vi "Hardware-EPTxControlCalPoints.vi"() -> (1 "EPTx Settings File Path":string, 3 "LoadEPTx Settings":bool, 4 "EPTxState":T4, 6 "EPTx Signal Select":T2, 8 "EPTxFilters":T3 {"Aux 4 [s]" format="%#_6p"; "Aux 3 [s]" format="%#_6p"; "Aux 2 [s]" format="%#_6p"; "Aux 1 [s]" format="%#_6p"; "Primary [s]" format="%#_6p"}, 10 "StallSpeed [RPM]":sgl, 15 "HistoryCAD":u8)   [LabVIEW 2016, in "DSI-RT.lvlib"]
uses:
  DSI-RT.lvlib
  <vilib>/Powertrain Controls/Device Drivers/Engine Position Tracking/EPTx/RevA/RT/Controls/EPTxState.ctl
  <vilib>/Powertrain Controls/Device Drivers/Engine Position Tracking/EPTx/RevA/RT/Controls/EPTxFilters.ctl
  <vilib>/Powertrain Controls/Device Drivers/DCM/Rev0/FPGA/Digital Channel.ctl
  <vilib>/addons/Software Calibration Management/xSCM/CalPoint.xnode
  <vilib>/Powertrain Controls/Device Drivers/Engine Position Tracking/EPTx/RevA/RT/EPTx - RevA - RT.lvlib
  <vilib>/Powertrain Controls/Device Drivers/DCM/Rev0/FPGA/DCM - FPGA.lvlib
  <vilib>/addons/Software Calibration Management/xSCM/ni_scm.dll
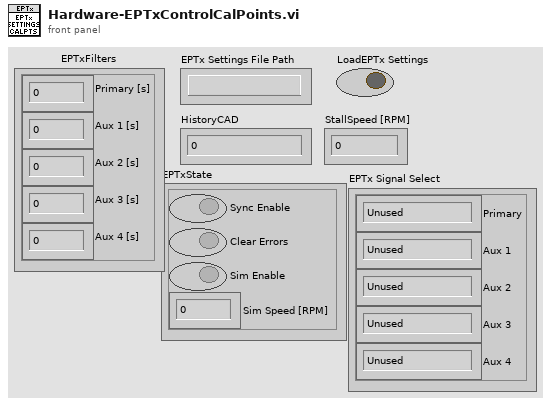
[diagram p1: front panel]
types:
  T1 = typedef "DCM - FPGA.lvlib/Digital Channel.ctl" = enum8{"Unused", "User OS", "Diff IO 1", "Diff IO 2", "Diff IO 3", "Diff IO 4", "Diff IO 5", "Diff IO 6", "Diff IO 7", "Diff IO 8", "Aux 1", "Aux 2", "Aux 3", "Aux 4", "Aux 5", "Aux 6", "Aux 7", "Aux 8", "Aux 9", "Aux 10", "Aux 11", "Aux 12", "Aux 13", "Aux 14", "Aux 15", "Aux 16"}
  T2 = cluster{"Primary":T1, "Aux 1":T1, "Aux 2":T1, "Aux 3":T1, "Aux 4":T1}
  T3 = typedef "EPTx - RevA - RT.lvlib/EPTxFilters.ctl" = cluster{"Primary [s]":sgl, "Aux 1 [s]":sgl, "Aux 2 [s]":sgl, "Aux 3 [s]":sgl, "Aux 4 [s]":sgl}
  T4 = typedef "EPTx - RevA - RT.lvlib/EPTxState.ctl" = cluster{"Sync Enable":bool, "Clear Errors":bool, "Sim Enable":bool, "Sim Speed [RPM]":sgl}
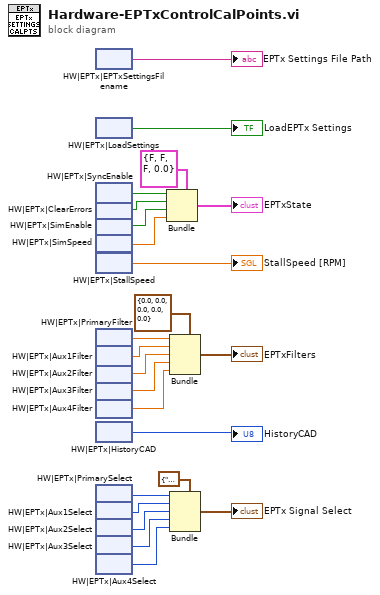
[diagram p0: block diagram]
diagram:
  n1 = xnode "HW|EPTx|EPTxSettingsFilename"() -> ("Value"=→"EPTx Settings File Path":string)
  n2 = xnode "HW|EPTx|LoadSettings"() -> ("Value"=→"LoadEPTx Settings":bool)
  n3 = xnode "HW|EPTx|SyncEnable"() -> ("Value"=w13:bool)
  n4 = xnode "HW|EPTx|ClearErrors"() -> ("Value"=w14:bool)
  n5 = xnode "HW|EPTx|SimEnable"() -> ("Value"=w15:bool)
  n6 = xnode "HW|EPTx|SimSpeed"() -> ("Value"=w16:sgl)
  n7 = xnode "HW|EPTx|StallSpeed"() -> ("Value"=→"StallSpeed [RPM]":sgl)
  n8 = xnode "HW|EPTx|PrimaryFilter"() -> ("Value"=w21:sgl)
  n9 = xnode "HW|EPTx|Aux1Filter"() -> ("Value"=w20:sgl)
  n10 = xnode "HW|EPTx|Aux2Filter"() -> ("Value"=w19:sgl)
  n11 = xnode "HW|EPTx|Aux3Filter"() -> ("Value"=w18:sgl)
  n12 = xnode "HW|EPTx|Aux4Filter"() -> ("Value"=w17:sgl)
  n13 = xnode "HW|EPTx|HistoryCAD"() -> ("Value"=→"HistoryCAD":u8)
  n14 = xnode "HW|EPTx|PrimarySelect"() -> ("Value"=w8:u8)
  n15 = xnode "HW|EPTx|Aux1Select"() -> ("Value"=w7:u8)
  n16 = xnode "HW|EPTx|Aux2Select"() -> ("Value"=w6:u8)
  n17 = xnode "HW|EPTx|Aux3Select"() -> ("Value"=w5:u8)
  n18 = xnode "HW|EPTx|Aux4Select"() -> ("Value"=w4:u8)
  n19 = Bundle(cluster=T4 {"Sync Enable"=FALSE, "Clear Errors"=FALSE, "Sim Enable"=FALSE, "Sim Speed [RPM]"=0.0} ("EPTxState 2"), "Sync Enable"=w13, "Clear Errors"=w14, "Sim Enable"=w15, "Sim Speed [RPM]"=w16) -> (→"EPTxState":T4)
  n20 = Bundle(cluster=T3 {"Primary [s]"=0.0, "Aux 1 [s]"=0.0, "Aux 2 [s]"=0.0, "Aux 3 [s]"=0.0, "Aux 4 [s]"=0.0} ("EPTxFilters"), "Primary [s]"=w21, "Aux 1 [s]"=w20, "Aux 2 [s]"=w19, "Aux 3 [s]"=w18, "Aux 4 [s]"=w17) -> (→"EPTxFilters":T3)
  n21 = Bundle(cluster=T2 {"Primary"=enum."Unused", "Aux 1"=enum."Unused", "Aux 2"=enum."Unused", "Aux 3"=enum."Unused", "Aux 4"=enum."Unused"} ("EPTx Signal Select"), "Primary"=w8, "Aux 1"=w7, "Aux 2"=w6, "Aux 3"=w5, "Aux 4"=w4) -> (→"EPTx Signal Select":T2)
